vi "Shoulder Position to Target Wrist Position.vi"(5 "Wrist Encoder Pos at 90 degrees":dbl, 7 "Min Wrist Encoder Pos":dbl, 8 "Shoulder Enc Position":dbl, 11 "Wanted Wrist Angle (-1,1)":dbl) -> (2 "Target Wrist Enc Position":dbl)   [LabVIEW 2023]
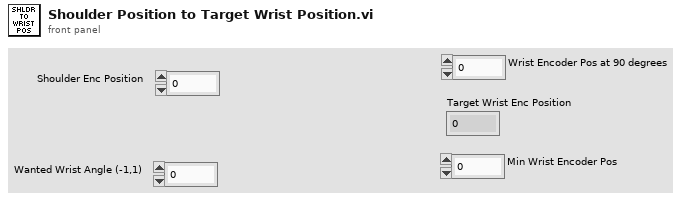
[diagram p1: front panel]
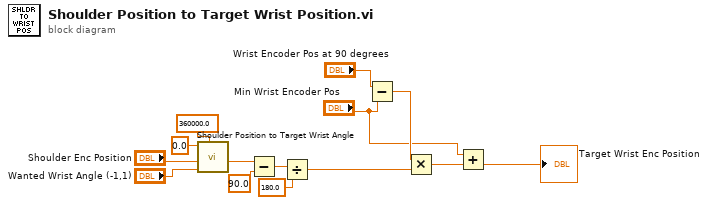
[diagram p0: block diagram]
diagram:
  n1 = call "Shoulder Position to Target Wrist Angle.vi"("Shoulder Max Enc"=360000.0, "Wanted Wrist Angle (-1, 1)"="Wanted Wrist Angle (-1,1)", "Shoulder Enc Positon"="Shoulder Enc Position", "Shoulder Min Enc"=0.0) -> ("Target Wrist Angle deg(90-270)"=w11:dbl)  [unwired: 7 in]
  n2 = Subtract(x=w11, y=90.0) -> (x-y=w9:dbl)
  n3 = Divide(x=w9, y=180.0) -> (x/y=w6:dbl)
  n4 = Subtract(x="Wrist Encoder Pos at 90 degrees", y="Min Wrist Encoder Pos") -> (x-y=w3:dbl)
  n5 = Multiply(x=w3, y=w6) -> (x*y=w7:dbl)
  n6 = Add(x="Min Wrist Encoder Pos", y=w7) -> (x+y=→"Target Wrist Enc Position":dbl)
